vi "Exchange VCH Parameters.vi"(8 "error in (no error)":errorcluster, 9 "PAR index":i32[](array[numeric]), 10 "Parameters":u32[](array[numeric])=[0, 10000, 5000, 1000, 0, 2], 11 "QM_VCH in":refnum<class "valve_VCH.lvclass">[](array[class])) -> (0 "error out":errorcluster, 3 "QM_VCH out":refnum<class "valve_VCH.lvclass">[](array[class]))   [LabVIEW 2019, in "valve_VCH.lvclass"]
uses:
  valve_VCH.lvclass
  valve_VCH.lvclass/valve_VCH.ctl
  Z_state/valve_VCH_Z_state.lvclass/valve_VCH_Z_state.ctl
  ZM_state/valve_VCH_ZM_state.lvclass/valve_VCH_ZM_state.ctl
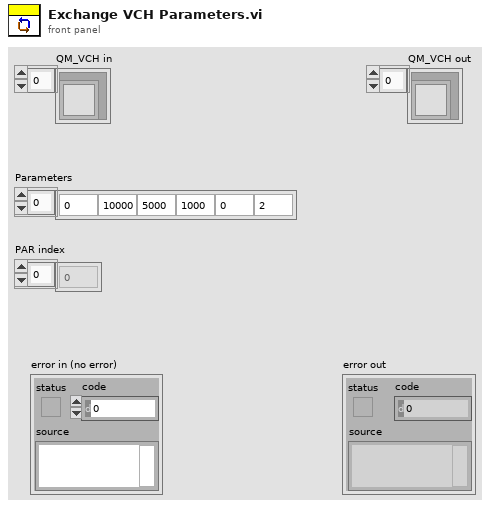
[diagram p1: front panel]
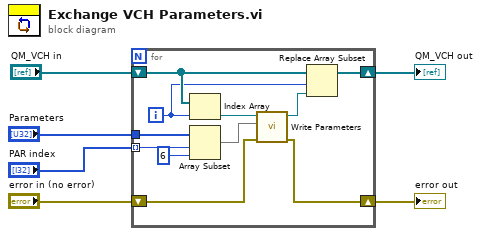
[diagram p0: block diagram]
diagram:
  n1 = for {
    shift-right: [w14] -> w1
    shift-left: "QM_VCH in" -> [w15]
    shift-right: [w12] -> w3
    shift-left: "error in (no error)" -> [w13]
    tunnel: "Parameters" -> [w11]
    tunnel: "PAR index" -> [w8] mode=indexing
    i -> [w7]
    n2 = Index Array(array=w15, index=w7) -> (element=w17:refnum<class "valve_VCH.lvclass">)
    n3 = Array Subset(array=w11, index=w8, length=6) -> (w10:u32[])
    n4 = call "Write Parameters.vi"("error in (no error)"=w13, "Parameters table VCH"=w10, "valve_VCH in"=w17) -> ("error out"=w12:errorcluster, "valve_VCH out"=w16:refnum<class "valve_VCH.lvclass">)  [unwired: 7 in]
    n5 = Replace Array Subset(array=w15, new element=w16, index=w7) -> (w14:refnum<class "valve_VCH.lvclass">[])
  }
  "error out" <- w3
  "QM_VCH out" <- w1
